vi "Joystick and Camera.vi"(11 "XYZTheta":dbl[](array[numeric])) -> (0 "error out":errorcluster, 1 "Gantry":dbl[](array[numeric]), 3 "Sum":dbl[](array[numeric]))   [LabVIEW 2016]
uses:
  Classes/Controllers/Camera/Copy of Camera Folder/Machine Vision.ctl
  Classes/Controllers/Motion/Copy of Motion Folder/Motion.lvclass
  Classes/Controllers/Camera/Copy of Controller Folder/Controller.lvclass
  Classes/Controllers/Camera/Copy of Camera Folder/Camera.lvclass
panel:
  out "Numeric 2":i32
  out "Numeric":dbl
  out "Image Out":T1(plugin-control)
  in  "Boolean":bool=TRUE
  in  "Go 2":bool
  in  "Z Go":bool
  in  "Position":dbl
  in  "Machine Vision":T2
  in  "Go":bool
  in  "Joystick":bool
  in  "Stop":bool
  out "Image":T1(plugin-control)
  out "Camera":dbl[](array[numeric])
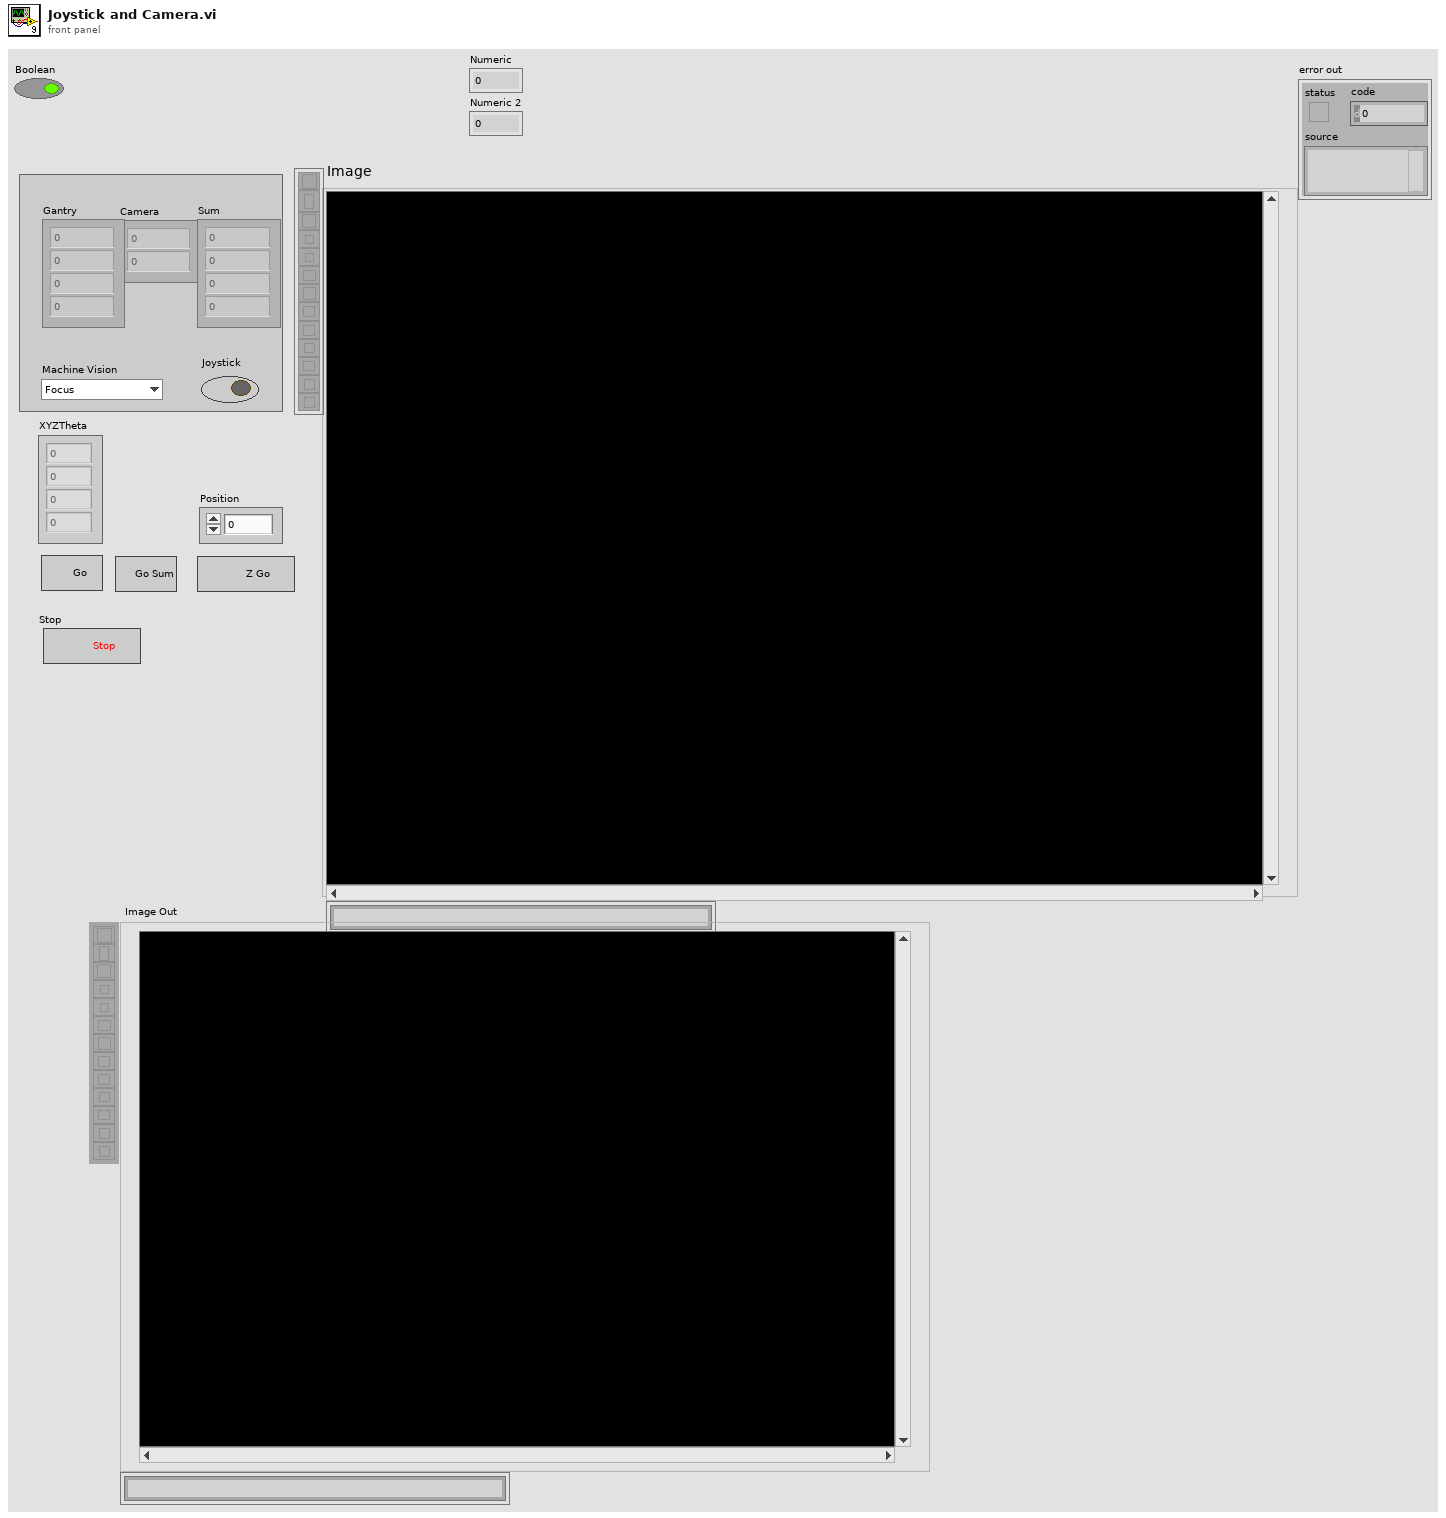
[diagram p1: front panel]
types:
  T1 = typedef "IMAQ Image.ctl" = refnum<image>
  T2 = typedef "Camera.lvclass/Machine Vision.ctl" = enum16{"Focus", "chip cross", "LargeCircle", "None", "INTT HDI Mark", "INTT Sensor Cross", "INTT Chip Corner", "HPK Silicon", "circle"}
  T3 = typedef "Controller.lvclass/Controllers.ctl" = cluster{"Copy of Motion.lvclass":refnum<class "Motion.lvclass">, "Copy of I-O.lvclass":refnum<class "I-O.lvclass">, "Copy of Dispenser.lvclass":refnum<class "Dispenser.lvclass">}
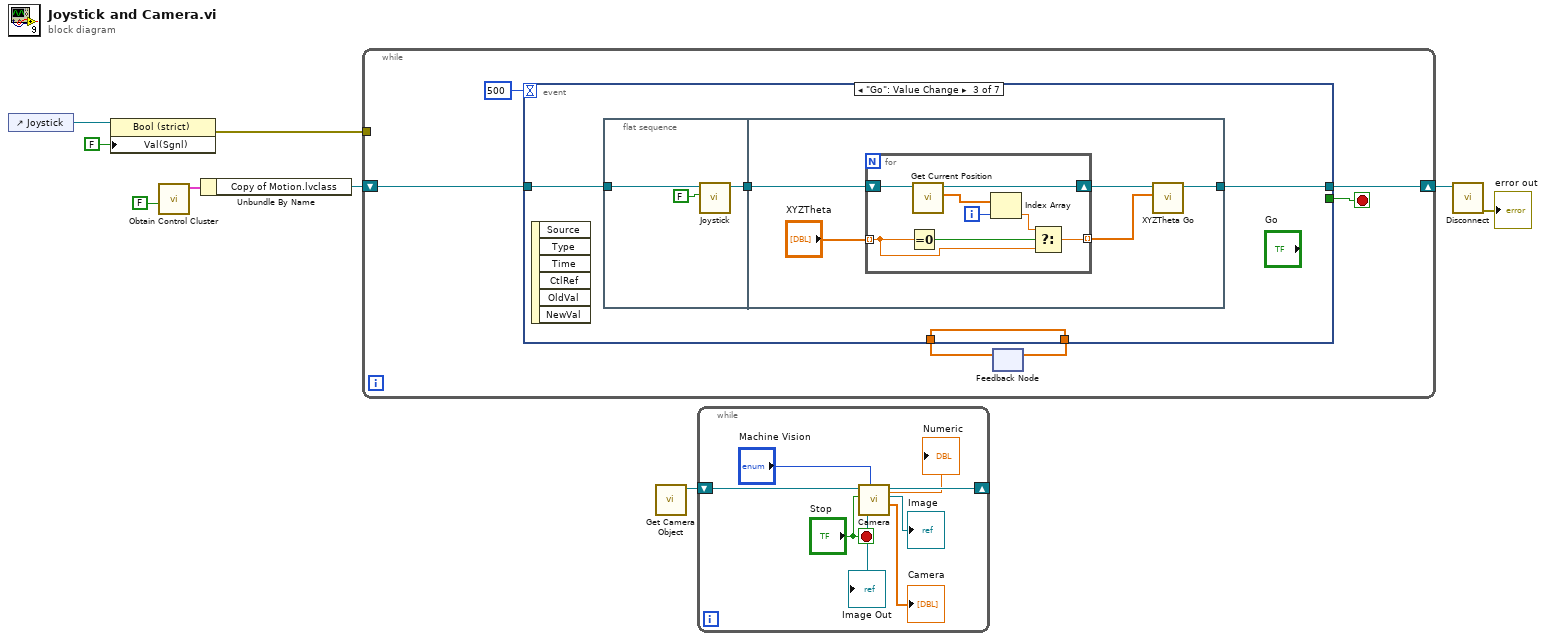
[diagram p0: block diagram]
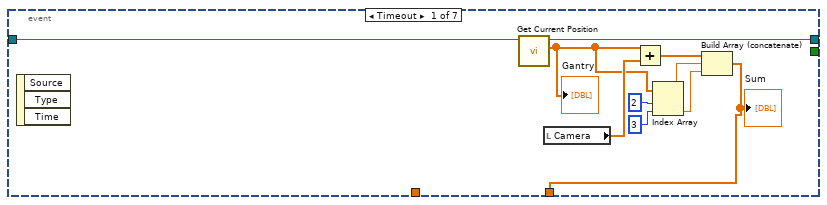
[diagram p2: hidden frame]
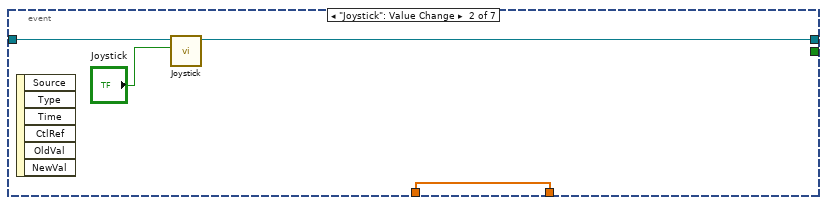
[diagram p3: hidden frame]
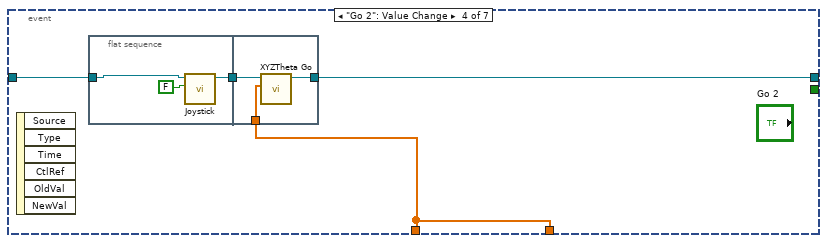
[diagram p4: hidden frame]
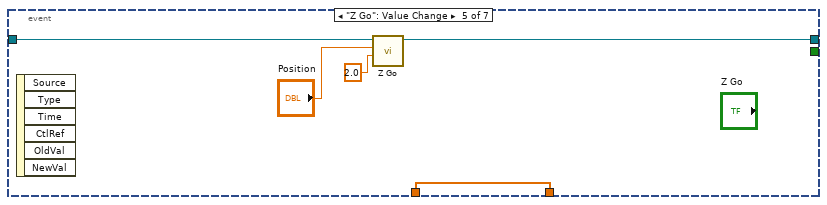
[diagram p5: hidden frame]
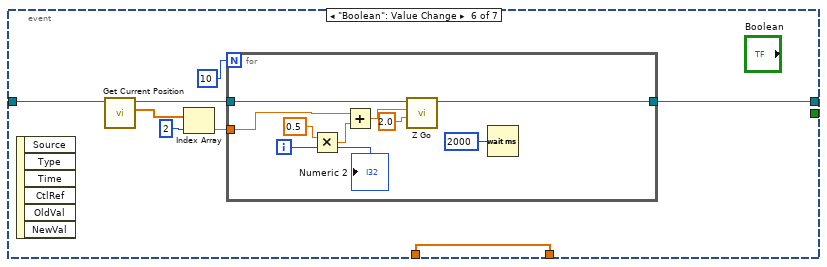
[diagram p6: hidden frame]
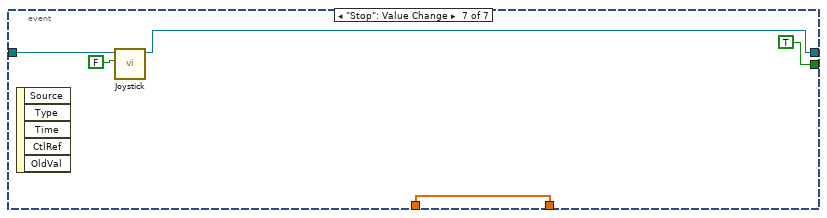
[diagram p7: hidden frame]
diagram:
  n1 = control-ref of="Joystick"() -> (w8:refnum<vi>)
  n2 = property class="Bool (strict)"(reference=w8, "Val(Sgnl)"=FALSE ("Value (Signaling)")) -> (error out=w6:errorcluster)  [unwired: 1 in, 1 out]
  n3 = call "Obtain Control Cluster.vi"("I/O"=FALSE) -> ("Control Out"=w4:T3)  [unwired: 10 in]
  n4 = Unbundle By Name(w4) -> ("Copy of Motion.lvclass"=w3:refnum<class "Motion.lvclass">)
  n5 = while {
    shift-right: [w10] -> w7
    shift-left: w3 -> [w13]
    tunnel: w6 -> [_]
    stop <- w14 stop-if-true
    n6 = feedback #1() -> (w11:dbl[])  [unwired: 1 in]
    n7 = event shown="[2] \"Go\": Value Change" {
      selector: _ -> [_ _ _ _ _ _ _]
      dyn-events: _ -> [_ _ _ _ _ _ _]
      timeout: 500 -> [_ _ _ _ _ _ _]
      tunnel: [_ _ _ _ _ _ TRUE] -> w14
      tunnel: w13 -> [w24 w29 w33 w53 w64 w72 w85]
      tunnel: [w23 w27 w32 w52 w63 w67 w83] -> w10
      tunnel: [w16 w26 w30 w50 w60 w65 w82] -> w12
      tunnel: w11 -> [_ w26 w30 w50 w60 w65 w82]
      event Timeout {
        n8 = event-data() -> ()  [unwired: 1 in, 3 out]
        n9 = call-dynamic "Get Current Position.vi"("Motion in"=w24) -> ("XYZTheta Out"=w21:dbl[], "Motion out"=w23:refnum<class "Motion.lvclass">)  [unwired: 8 in, 1 out]
        "Gantry" <- w21
        n10 = local read "Camera"() -> (w25:dbl[])
        n11 = Add(x=w21, y=w25) -> (x+y=w22:dbl[])
        n12 = Index Array(array=w21, index #1=2 ("index"), index #2=3 ("index")) -> (element #1=w18:dbl, element #2=w17:dbl)
        n13 = Build Array (concatenate)(w22, w18, w17) -> (w16:dbl[])
        "Sum" <- w16
      }
      event "Joystick": Value Change {
        n14 = event-data() -> ()  [unwired: 1 in, 6 out]
        n15 = call-dynamic "Joystick.vi"("Joystick"="Joystick", "Motion in"=w29) -> ("Motion out"=w27:refnum<class "Motion.lvclass">)  [unwired: 8 in, 1 out]
      }
      event "Go": Value Change {
        n16 = event-data() -> ()  [unwired: 1 in, 6 out]
        n17 = flat-sequence {
          tunnel: w33 -> [w35]
          tunnel: [w34] -> w31
          tunnel: [w37] -> w32
          tunnel: w31 -> [w40]
          frame #0 {
            n18 = call-dynamic "Joystick.vi"("Joystick"=FALSE, "Motion in"=w35) -> ("Motion out"=w34:refnum<class "Motion.lvclass">)  [unwired: 8 in, 1 out]
          }
          frame #1 {
            n19 = for {
              tunnel: "XYZTheta" -> [w47] mode=indexing
              tunnel: [w45] -> w39 mode=indexing
              shift-right: [w43] -> w38
              shift-left: w40 -> [w44]
              i -> [w49]
              n20 = Equal To 0?(x=w47) -> (x = 0?=w48:bool)
              n21 = call-dynamic "Get Current Position.vi"("Motion in"=w44) -> ("XYZTheta Out"=w42:dbl[], "Motion out"=w43:refnum<class "Motion.lvclass">)  [unwired: 8 in, 1 out]
              n22 = Index Array(array=w42, index=w49) -> (element=w46:dbl)
              n23 = Select(t=w46, s=w48, f=w47) -> (s? t:f=w45:dbl)
            }
            n24 = call "XYZTheta Go.vi"("XYZTheta In"=w39, "Motion in"=w38) -> ("Motion out"=w37:refnum<class "Motion.lvclass">)  [unwired: 7 in, 2 out]
          }
        }
      }
      event "Go 2": Value Change {
        n25 = event-data() -> ()  [unwired: 1 in, 6 out]
        n26 = flat-sequence {
          tunnel: w53 -> [w55]
          tunnel: [w54] -> w51
          tunnel: [w59] -> w52
          tunnel: w51 -> [w58]
          tunnel: w50 -> [w57]
          frame #0 {
            n27 = call-dynamic "Joystick.vi"("Joystick"=FALSE, "Motion in"=w55) -> ("Motion out"=w54:refnum<class "Motion.lvclass">)  [unwired: 8 in, 1 out]
          }
          frame #1 {
            n28 = call "XYZTheta Go.vi"("XYZTheta In"=w57, "Motion in"=w58) -> ("Motion out"=w59:refnum<class "Motion.lvclass">)  [unwired: 7 in, 2 out]
          }
        }
      }
      event "Z Go": Value Change {
        n29 = event-data() -> ()  [unwired: 1 in, 6 out]
        n30 = call-dynamic "Z Go.vi"("Speed"=2.0, "Position"="Position", "Motion in"=w64) -> ("Motion out"=w63:refnum<class "Motion.lvclass">)  [unwired: 7 in, 1 out]
      }
      event "Boolean": Value Change {
        n31 = event-data() -> ()  [unwired: 1 in, 6 out]
        n32 = call-dynamic "Get Current Position.vi"("Motion in"=w72) -> ("XYZTheta Out"=w70:dbl[], "Motion out"=w71:refnum<class "Motion.lvclass">)  [unwired: 8 in, 1 out]
        n33 = Index Array(array=w70, index=2) -> (element=w68:dbl)
        n34 = for {
          N: 10 -> [_]
          tunnel: w71 -> [w80]
          tunnel: w68 -> [w76]
          tunnel: [w74] -> w67
          i -> [w79]
          n35 = Multiply(x=0.5, y=w79) -> (x*y=w77:dbl)
          n36 = Add(x=w76, y=w77) -> (x+y=w75:dbl)
          n37 = call-dynamic "Z Go.vi"("Speed"=2.0, "Position"=w75, "Motion in"=w80) -> ("Motion out"=w74:refnum<class "Motion.lvclass">)  [unwired: 7 in, 1 out]
          n38 = Wait (ms)(milliseconds to wait=u32 2000) -> ()  [unwired: 1 out]
          "Numeric 2" <- w79
        }
      }
      event "Stop": Value Change {
        n39 = event-data() -> ()  [unwired: 1 in, 5 out]
        n40 = call-dynamic "Joystick.vi"("Joystick"=FALSE, "Motion in"=w85) -> ("Motion out"=w83:refnum<class "Motion.lvclass">)  [unwired: 8 in, 1 out]
      }
    }
    n41 = feedback-in #1(w12) -> ()
  }
  n42 = call "Get Camera Object.vi"() -> ("Camera out"=w2:refnum<class "Camera.lvclass">)  [unwired: 10 in, 1 out]
  n43 = while {
    shift-right: [w93] -> _
    shift-left: w2 -> [w94]
    stop <- "Stop" stop-if-true
    n44 = call "Camera.vi"("Machine Vision"="Machine Vision", "Stop"="Stop", "Camera in"=w94) -> ("Camera"=→"Camera":dbl[], "Image"=→"Image":T1, "Camera out"=w93:refnum<class "Camera.lvclass">, "Image Out"=→"Image Out":T1, "Numeric"=→"Numeric":dbl)  [unwired: 2 in, 2 out]
  }
  n45 = call-dynamic "Disconnect.vi"("Controller in"=w7) -> ("error out"=→"error out":errorcluster)  [unwired: 9 in]
